vi "getRange.vi"(8 "error in (no error)":errorcluster, 11 "DmmKeysight in":refnum<class "DmmKeysight.lvclass">) -> (0 "error out":errorcluster, 2 "range":dbl, 3 "DmmKeysight out":refnum<class "DmmKeysight.lvclass">)   [LabVIEW 2023, in "DmmKeysight.lvclass"]
doc: "<b>Author:</b> Wolfgang\n<b>Description:</b> return measurement range of the dmm based for the actual selected mode"
uses:
  DmmKeysight.lvclass
  DmmKeysight.lvclass/DmmKeysight.ctl
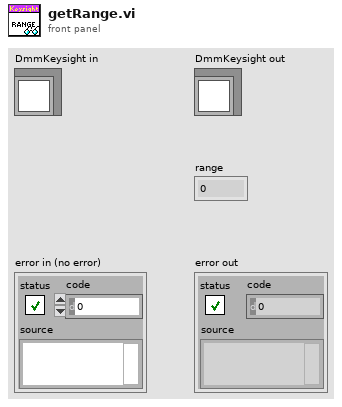
[diagram p1: front panel]
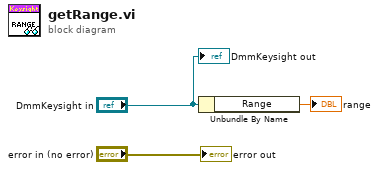
[diagram p0: block diagram]
diagram:
  n1 = Unbundle By Name("DmmKeysight in") -> ("Range"=→"range":dbl)
  "error out" <- "error in (no error)"
  "DmmKeysight out" <- "DmmKeysight in"
